vi "rad_Deploy Image Wrapper.vi"(4 "Deploy":string[](array[string]), 6 "restart after imaging (T)":bool=TRUE, 7 "Deployment Notifiers":T3, 8 "error in (no error)":errorcluster, 9 "apply primary NIC from image (F)":bool, 10 "image file path":path, 11 "Target settings in":T1={"Hostname"="", "Serial number"="", "Product name"="", "Product code"=0, "System status"="", "Credential type"=enum."None/Unlocked", "User added?"=FALSE, "Primary NIC"={"MAC address"="", "IP Address Request Mode"=2, "IP address"="", "Subnet mask"="", "Gateway"="", "DNS server"=""}} {"Primary NIC"."IP Address Request Mode" items=["Static"=1, "DHCP/Link-Local"=2, "Link-Local Only"=4, "DHCP Only"=8]}) -> (0 "error out":errorcluster, 2 "image file path":path, 3 "Target settings out":T1={"Hostname"="", "Serial number"="", "Product name"="", "Product code"=0, "System status"="", "Credential type"=enum."None/Unlocked", "User added?"=FALSE, "Primary NIC"={"MAC address"="", "IP Address Request Mode"=2, "IP address"="", "Subnet mask"="", "Gateway"="", "DNS server"=""}} {"Primary NIC"."IP Address Request Mode" items=["Static"=1, "DHCP/Link-Local"=2, "Link-Local Only"=4, "DHCP Only"=8]})   [LabVIEW 2016]
uses:
  TypeDefs/rad_Deployment Notifiers.ctl
  TypeDefs/rad_Deployment Status Data Type.ctl
  TypeDefs/rad_Deployment Progress Data Type.ctl
  Targets/TypeDefs/rad_Target Information.ctl
  Targets/TypeDefs/rad_Target Network Settings.ctl
  <vilib>/nisyscfg/Network Settings Image.ctl
  <vilib>/nisyscfg/Set System Image (Folder).vi
  <vilib>/nisyscfg/Close (System).vi
  <vilib>/nisyscfg/nisyscfg.lvlib
panel:
  out "finished":bool
  in  "Stop Checking for Events":bool
  out "Progress":u8(slide) scale=0.0..100.0
  out "Status":string
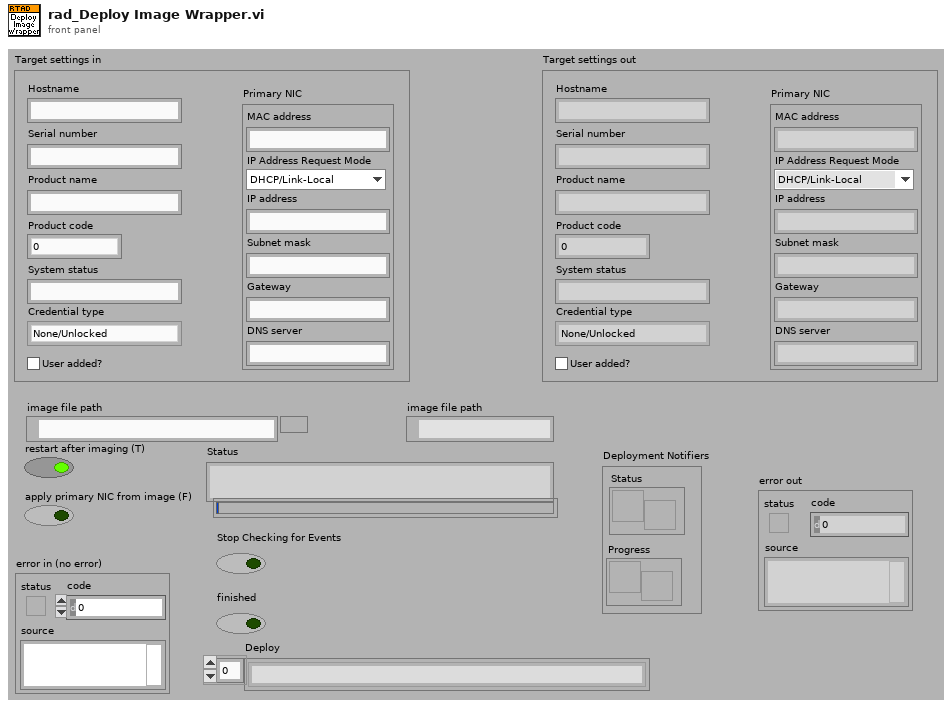
[diagram p1: front panel]
types:
  T1 = typedef "rad_Target Information.ctl" = cluster{"Hostname":string, "Serial number":string, "Product name":string, "Product code":i32, "System status":string, "Credential type":enum16{"None/Unlocked", "FTP Password", "NIAuth Credentials"}, "User added?":bool, "Primary NIC":T2}
  T2 = typedef "rad_Target Network Settings.ctl" = cluster{"MAC address":string, "IP Address Request Mode":i32, "IP address":string, "Subnet mask":string, "Gateway":string, "DNS server":string}
  T3 = typedef "rad_Deployment Notifiers.ctl" = cluster{"Status":refnum<notifier>, "Progress":refnum<notifier>}
  T4 = typedef "rad_Deployment Progress Data Type.ctl" = i8
  T5 = typedef "nisyscfg.lvlib/Network Settings Image.ctl" = u32
  T6 = enum32{"state changed", "beginning restart", "getting file", "putting file", "creating directory", "deleting file", "deleting directory", "enumerating file system", "renaming file", "current component", "operation progress", "downloading file", "unpacking file", "running install script"}
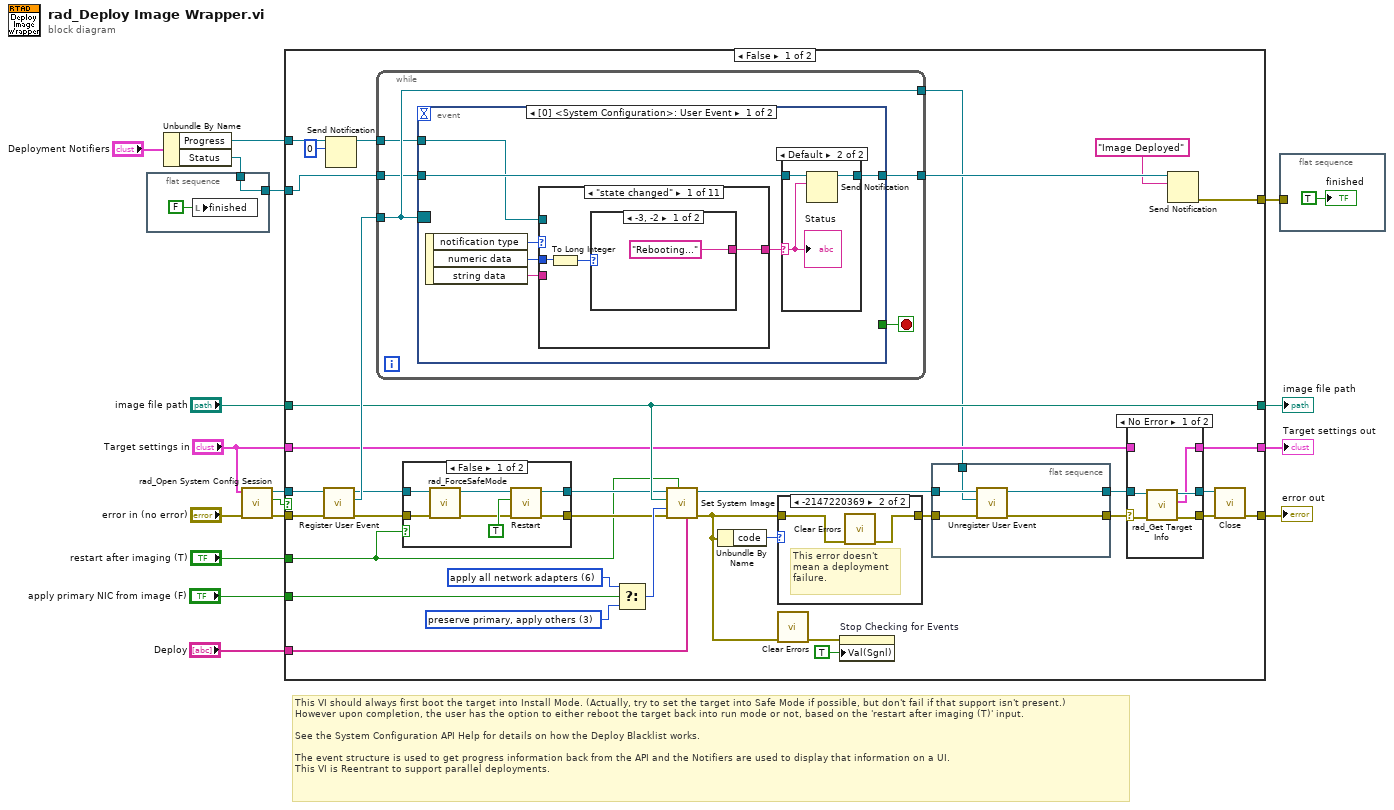
[diagram p0: block diagram]
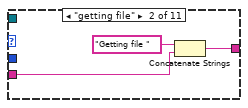
[diagram p7: hidden frame]
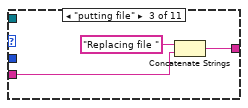
[diagram p8: hidden frame]
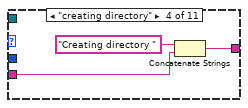
[diagram p9: hidden frame]
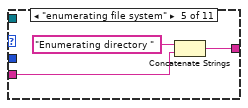
[diagram p10: hidden frame]
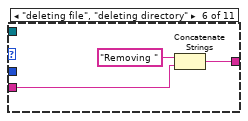
[diagram p11: hidden frame]
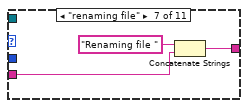
[diagram p12: hidden frame]
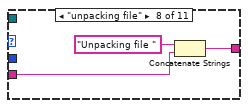
[diagram p13: hidden frame]
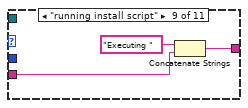
[diagram p14: hidden frame]
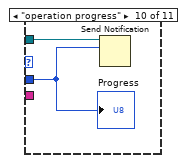
[diagram p15: hidden frame]
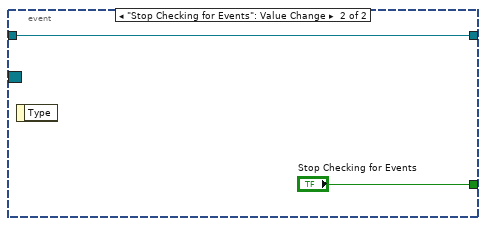
[diagram p17: hidden frame]
diagram:
  # "This VI should always first boot the target into Install Mode. (Actually, try to set the target into Safe Mode if possible, but don't fail if that support isn't present.)\nHowever upon completion, the user has the option to either reboot the target back into run mode or not, based on the 'restart after imaging (T)' input.\n\nSee the System Configuration API Help for details on how the Deploy Blacklist works.\n\nThe event structure is used to get progress information back from the API and the Notifiers are used to display that information on a UI. \nThis VI is Reentrant to support parallel deployments."
  n1 = flat-sequence {
    tunnel: [w18] -> w3
    tunnel: w2 -> [w18]
    frame #0 {
      n2 = local write "finished"(FALSE ("finished")) -> ()
    }
  }
  n3 = Unbundle By Name("Deployment Notifiers") -> ("Progress"=w11:refnum<notifier>, "Status"=w2:refnum<notifier>)
  n4 = call "rad_Open System Config Session.vi"("error in (no error)"="error in (no error)", "Target settings"="Target settings in") -> ("error out"=w7:errorcluster, "Cancelled"=w6:bool, "Session out"=w8:refnum<k21>)  [unwired: 6 in, 1 out]
  n5 = case shown="False" w6 {
    tunnel: [w54 w130] -> w17
    tunnel: "image file path" -> [w40 w129]
    tunnel: "restart after imaging (T)" -> [w32 _]
    tunnel: w8 -> [w53 _]
    tunnel: w7 -> [w52 w130]
    tunnel: [w48 _] -> w14
    tunnel: "apply primary NIC from image (F)" -> [w47 _]
    tunnel: w11 -> [w43 _]
    tunnel: [w40 w129] -> w16
    tunnel: "Deploy" -> [w39 _]
    tunnel: "Target settings in" -> [w28 w128]
    tunnel: [w29 w128] -> w4
    tunnel: w3 -> [w23 _]
    frame False {
      w46 = T5 6 items=["reset primary, disable others", "preserve primary, disable others", "preserve all network adapters", "preserve primary, apply others", "apply primary, disable others", "apply primary, preserve others", "apply all network adapters"] ("network settings (apply all adapters)")
      w45 = T5 3 items=["reset primary, disable others", "preserve primary, disable others", "preserve all network adapters", "preserve primary, apply others", "apply primary, disable others", "apply primary, preserve others", "apply all network adapters"] ("network settings (apply all adapters)")
      n6 = call <vilib>:"Register User Event.vi"("error in (no error)"=w52, "Session in"=w53) -> ("error out"=w35:errorcluster, "Event Registration out"=w51:refnum<event-registration>, "Session out"=w36:refnum<k21>)  [unwired: 7 in]
      n7 = Send Notification(notification=T4 0, notifier=w43) -> (notifier out=w42:refnum<notifier>)  [unwired: 1 in, 1 out]
      n8 = while {
        tunnel: w51 -> [w84]
        tunnel: [w84] -> w26
        tunnel: w23 -> [w82]
        tunnel: [w81] -> w50
        tunnel: w42 -> [w80]
        stop <- w83 stop-if-true
        n9 = event shown="[0] <System Configuration>: User Event" {
          selector: w84 -> [_ _]
          dyn-events: _ -> [_ _]
          timeout: _ -> [_ _]
          tunnel: [_ "Stop Checking for Events"] -> w83
          tunnel: w82 -> [w87 w126]
          tunnel: [w86 w126] -> w81
          tunnel: w80 -> [w85 _]
          event User Event {
            n10 = event-data() -> ("notification type"=w91:T6, "numeric data"=w89:u32, "string data"=w90:string)  [unwired: 1 in]
            n11 = case shown="\"state changed\"" w91 {
              tunnel: [w96 w100 w103 w106 w109 w112 w115 w118 w121 _ _] -> w88
              tunnel: w90 -> [_ w101 w104 w107 w110 w113 w116 w119 w122 _ _]
              tunnel: w89 -> [w98 _ _ _ _ _ _ _ _ w125 _]
              tunnel: w85 -> [_ _ _ _ _ _ _ _ _ w124 _]
              frame "state changed" {
                n12 = To Long Integer(number=w98) -> (32bit integer=w97:i32)
                n13 = case shown="-3, -2" w97 {
                  tunnel: ["Rebooting..." _] -> w96
                  frame -3, -2 {
                  }
                  frame Default {
                  }
                }
              }
              frame "getting file" {
                n14 = Concatenate Strings("Getting file " ("Status"), w101) -> (w100:string)
              }
              frame "putting file" {
                n15 = Concatenate Strings("Replacing file " ("Status"), w104) -> (w103:string)
              }
              frame "creating directory" {
                n16 = Concatenate Strings("Creating directory " ("Status"), w107) -> (w106:string)
              }
              frame "enumerating file system" {
                n17 = Concatenate Strings("Enumerating directory " ("Status"), w110) -> (w109:string)
              }
              frame "deleting file", "deleting directory" {
                n18 = Concatenate Strings("Removing " ("Status"), w113) -> (w112:string)
              }
              frame "renaming file" {
                n19 = Concatenate Strings("Renaming file " ("Status"), w116) -> (w115:string)
              }
              frame "unpacking file" {
                n20 = Concatenate Strings("Unpacking file " ("Status"), w119) -> (w118:string)
              }
              frame "running install script" {
                n21 = Concatenate Strings("Executing " ("Status"), w122) -> (w121:string)
              }
              frame "operation progress" {
                n22 = Send Notification(notification=w125, notifier=w124) -> ()  [unwired: 1 in, 2 out]
                "Progress" <- w125
              }
              frame Default {
              }
            }
            n23 = case shown="Default" w88 {
              selector: w88 -> [_ w94]
              tunnel: w87 -> [w92 w95]
              tunnel: [w92 w93] -> w86
              frame "" {
              }
              frame Default {
                n24 = Send Notification(notification=w94, notifier=w95) -> (notifier out=w93:refnum<notifier>)  [unwired: 1 in, 1 out]
                "Status" <- w94
              }
            }
          }
          event "Stop Checking for Events": Value Change {
            n25 = event-data() -> ()  [unwired: 1 in, 1 out]
          }
        }
      }
      n26 = case shown="False" w32 {
        tunnel: w36 -> [w69 w71]
        tunnel: w35 -> [w64 w70]
        tunnel: [w67 w71] -> w34
        tunnel: [w66 w70] -> w33
        frame False {
          n27 = call "rad_ForceSafeMode.vi"("error in (no error)"=w64, "Target in"=w69) -> ("error out"=w63:errorcluster, "Target out"=w65:refnum<k21>)  [unwired: 8 in]
          n28 = call <vilib>:"Restart.vi"("error in (no error)"=w63, "Install Mode (F)"=TRUE ("install mode (F)"), "Session in"=w65) -> ("error out"=w66:errorcluster, "Session out"=w67:refnum<k21>)  [unwired: 6 in, 1 out]
        }
        frame True {
        }
      }
      n29 = Select(t=w46, s=w47, f=w45) -> (s? t:f=w44:T5)
      n30 = call-poly <vilib>:"Set System Image.vi"("File and Directory Blacklist"=w39, "Restart Automatically (T)"=w32, "error in (no error)"=w33, "Network Settings (preserve primary adapter, apply others)"=w44, "Source Folder"=w40, "Session in"=w34) -> ("error out"=w21:errorcluster, "Session out"=w27:refnum<k21>)  [unwired: 4 in]
      n31 = Unbundle By Name(w21) -> ("code"=w38:i32)
      n32 = case shown="-2147220369" w38 {
        tunnel: w21 -> [w72 w74]
        tunnel: [w72 w73] -> w37
        frame Default {
        }
        frame -2147220369 {
          # "This error doesn't\nmean a deployment\nfailure."
          n33 = call <vilib>:"Clear Errors.vi"("error in (no error)"=w74) -> ("error out"=w73:errorcluster)  [unwired: 5 in, 1 out]
        }
      }
      n34 = call <vilib>:"Clear Errors.vi"("error in (no error)"=w21) -> ("error out"=w20:errorcluster)  [unwired: 5 in, 1 out]
      n35 = property on="Stop Checking for Events" class="Bool (strict)"(error in=w20, "Val(Sgnl)"=TRUE ("Stop Checking for Events")) -> ()  [unwired: 1 in, 2 out]
      n36 = flat-sequence {
        tunnel: w37 -> [w79]
        tunnel: w27 -> [w78]
        tunnel: w26 -> [w77]
        tunnel: [w76] -> w25
        tunnel: [w75] -> w24
        frame #0 {
          n37 = call <vilib>:"Unregister User Event.vi"("error in (no error)"=w79, "Event Registration in"=w77, "Session in"=w78) -> ("error out"=w76:errorcluster, "Session out"=w75:refnum<k21>)  [unwired: 7 in]
        }
      }
      n38 = case shown="No Error" w25 {
        selector: w25 -> [w58 w62]
        tunnel: [w56 w62] -> w31
        tunnel: w24 -> [w59 w61]
        tunnel: [w57 w61] -> w30
        tunnel: [w55 w60] -> w29
        tunnel: w28 -> [_ w60]
        frame No Error {
          n39 = call "rad_Get Target Info.vi"("error in (no error)"=w58, "System Session in"=w59) -> ("error out"=w56:errorcluster, "Target settings"=w55:T1, "System Session out"=w57:refnum<k21>)  [unwired: 7 in]
        }
        frame Error {
        }
      }
      n40 = Send Notification(notification="Image Deployed", notifier=w50) -> (error out=w48:errorcluster)  [unwired: 1 in, 1 out]
      n41 = call-poly <vilib>:"Close.vi"("error in (no error)"=w31, "Session in"=w30) -> ("error out"=w54:errorcluster)  [unwired: 9 in]
    }
    frame True {
    }
  }
  "error out" <- w17
  "image file path" <- w16
  "Target settings out" <- w4
  n42 = flat-sequence {
    tunnel: w14 -> [_]
    frame #0 {
      "finished" <- TRUE ("finished")
    }
  }
